vi "Read all from stderr.vi"(11 "subprocess in":refnum<class "Buffered Subprocess.lvclass">) -> (2 "data":refnum<class "Bytestream.lvclass">, 3 "subprocess out":refnum<class "Buffered Subprocess.lvclass">)   [LabVIEW 2020, in "NI_Subprocess.lvlib" / "Buffered Subprocess.lvclass"]
uses:
  <vilib>/Subprocess/Buffered Subprocess/Buffered Subprocess.lvclass
  <vilib>/Array/Bytestream/Bytestream.lvclass
  <vilib>/Subprocess/Buffered Subprocess/Buffered Subprocess.lvclass/Buffered Subprocess.ctl
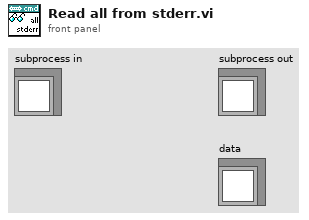
[diagram p1: front panel]
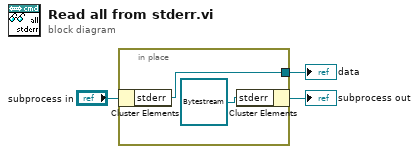
[diagram p0: block diagram]
diagram:
  n1 = in-place {
    in-place-border: [w5] -> w2
    n2 = in-place-cluster #1("subprocess in") -> ("stderr"=w5:refnum<class "Bytestream.lvclass">)
    n3 = in-place-cluster #1("stderr"=refnum<class "Bytestream.lvclass"> refnum) -> (→"subprocess out":refnum<class "Buffered Subprocess.lvclass">)
  }
  "data" <- w2
